vi "Tree - Populate.vi"(6 "Item Values":string[][](array[string]), 8 "error in (no error)":errorcluster, 9 "Item Indentation":i32[](array[numeric]), 10 "Item Names":string[](array[string]), 11 "TreeControl in":refnum<vi>) -> (0 "error out":errorcluster, 3 "TreeControl out":refnum<vi>)   [LabVIEW 2020]
panel:
  in  "Open All ?":bool
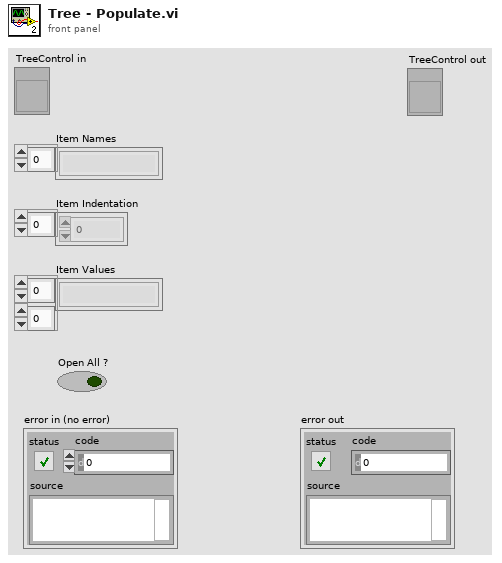
[diagram p1: front panel]
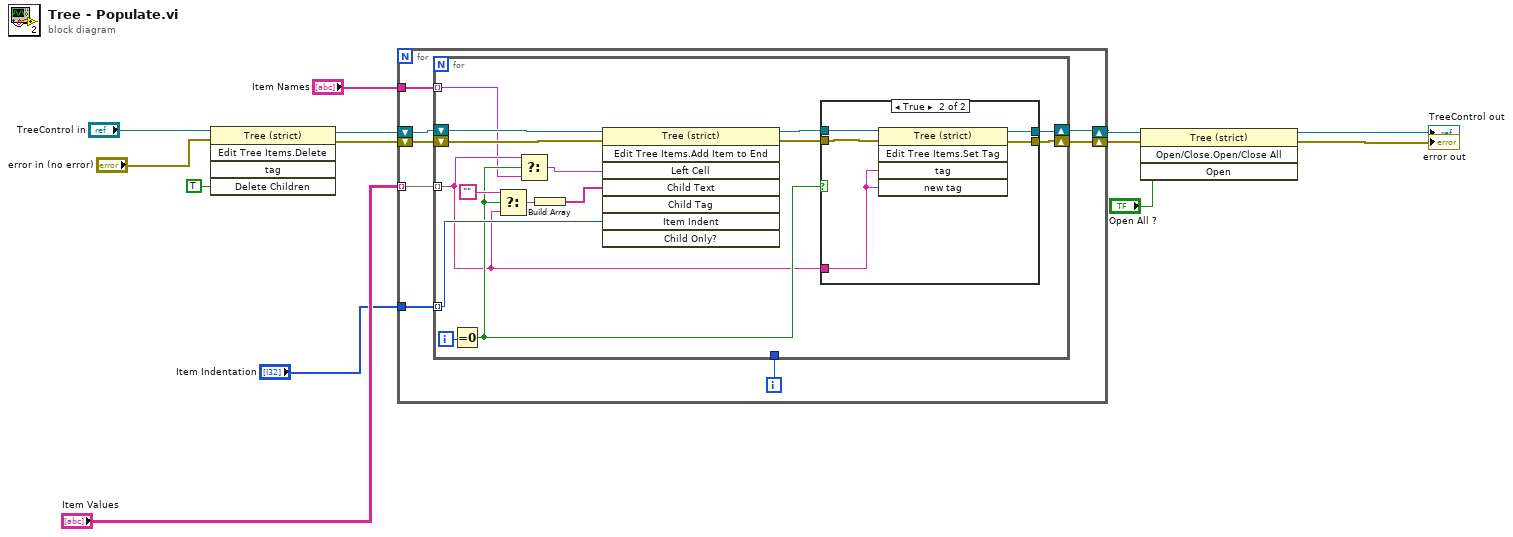
[diagram p0: block diagram]
diagram:
  n1 = invoke class="Tree (strict)" method="Edit Tree Items.Delete"(reference="TreeControl in", error in="error in (no error)", "Delete Children"=TRUE ("Delete Children?")) -> (reference out=w5:refnum<vi>, error out=w4:errorcluster)  [unwired: 2 in, 3 out]
  n2 = for {
    shift-right: [w18] -> w9
    shift-left: w4 -> [w20]
    shift-right: [w19] -> w10
    shift-left: w5 -> [w21]
    tunnel: "Item Indentation" -> [w17]
    tunnel: "Item Names" -> [w16]
    tunnel: "Item Values" -> [w15] mode=indexing
    i -> [w14]
    n3 = for {
      tunnel: w17 -> [w34] mode=indexing
      tunnel: w16 -> [w23] mode=indexing
      shift-right: [w31] -> w19
      shift-left: w21 -> [w36]
      shift-right: [w29] -> w18
      shift-left: w20 -> [w35]
      tunnel: w15 -> [w24] mode=indexing
      tunnel: w14 -> [_]
      i -> [w28]
      n4 = Equal To 0?(x=w28) -> (x = 0?=w25:bool)
      n5 = Select(t="", s=w25, f=w24) -> (s? t:f=w26:string)
      n6 = Select(t=w24, s=w25, f=w23) -> (s? t:f=w22:string)
      n7 = Build Array(w26) -> (w33:string[])
      n8 = invoke class="Tree (strict)" method="Edit Tree Items.Add Item to End"(reference=w36, error in=w35, "Left Cell"=w22, "Child Text"=w33, "Item Indent"=w34) -> (reference out=w32:refnum<vi>, error out=w30:errorcluster)  [unwired: 3 in, 6 out]
      n9 = case shown="True" w25 {
        tunnel: w32 -> [w38 w43]
        tunnel: [w38 w42] -> w31
        tunnel: w30 -> [w37 w41]
        tunnel: [w37 w40] -> w29
        tunnel: w24 -> [_ w39]
        frame False {
        }
        frame True {
          n10 = invoke class="Tree (strict)" method="Edit Tree Items.Set Tag"(reference=w43, error in=w41, "tag"=w39, "new tag"=w39) -> (reference out=w42:refnum<vi>, error out=w40:errorcluster)  [unwired: 1 in, 3 out]
        }
      }
    }
  }
  n11 = invoke class="Tree (strict)" method="Open/Close.Open/Close All"(reference=w10, error in=w9, "Open"="Open All ?") -> (reference out=→"TreeControl out":refnum<vi>, error out=→"error out":errorcluster)  [unwired: 1 in, 2 out]
